vi "ObjectRegistration.vi"(6 "Min Size":i32=40, 7 "Threshold":i32=30, 8 "error in (no error)":errorcluster, 10 "Roy":T1, 11 "Rob":T1) -> (0 "error out":errorcluster, 1 "Alignment quality":dbl, 2 "y displacement":dbl, 3 "x displacement":dbl)   [LabVIEW 2012]
uses:
  <vilib>/vision/Image Controls.llb/IMAQ Image.ctl
panel:
  out "Roy 2":T1(plugin-control)
  out "Roy":T1(plugin-control)
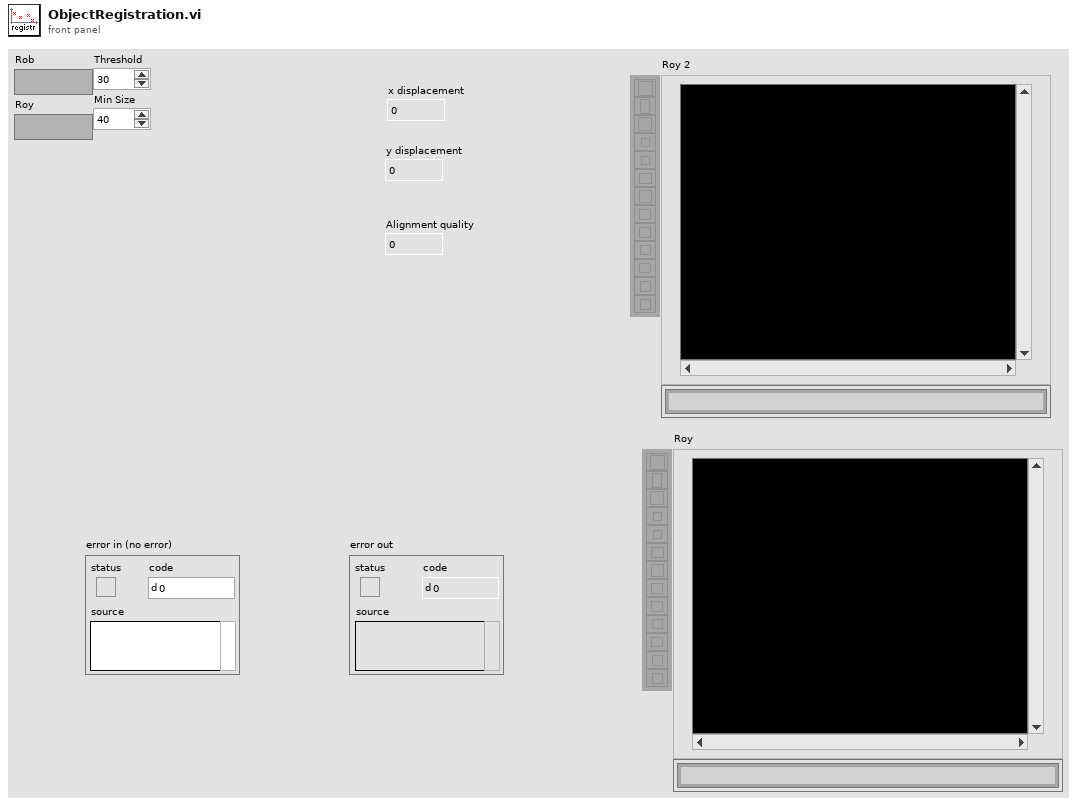
[diagram p1: front panel]
types:
  T1 = typedef "IMAQ Image.ctl" = refnum<image>
  T2 = cluster{"Objects":u16, "Threshold":i32, "Reject Border":bool, "Fill Holes":bool, "Min Object Size":bool, "Min Size":i32, "Max Object Size":bool, "Max Size":i32, "Show Search Area":bool, "Show Center":bool, "Show Bounding Box":bool}
  T3 = cluster{"Object Center":cluster{"X":sgl, "Y":sgl}, "Bounding Box":cluster{"X Left":i32, "Y Top":i32, "X Right":i32, "Y Bottom":i32}, "Area":sgl, "Orientation":sgl, "Aspect Ratio":sgl, "Nb Holes":i32}[]
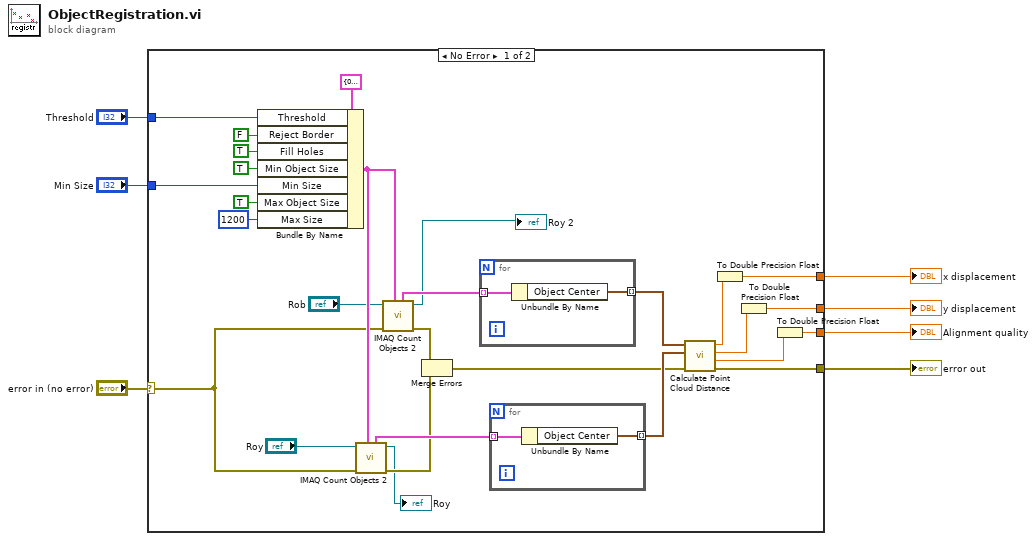
[diagram p0: block diagram]
diagram:
  n1 = case shown="No Error" "error in (no error)" {
    selector: "error in (no error)" -> [w21 w40]
    tunnel: [w20 w40] -> w6
    tunnel: [w16 _] -> w5
    tunnel: [w15 _] -> w4
    tunnel: [w14 _] -> w3
    tunnel: "Threshold" -> [w11 _]
    tunnel: "Min Size" -> [w10 _]
    frame No Error {
      n2 = Bundle By Name(cluster=T2 {"Objects"=0, "Threshold"=128, "Reject Border"=FALSE, "Fill Holes"=FALSE, "Min Object Size"=FALSE, "Min Size"=3, "Max Object Size"=FALSE, "Max Size"=100, "Show Search Area"=FALSE, "Show Center"=TRUE, "Show Bounding Box"=TRUE} ("Settings"), "Threshold"=w11, "Reject Border"=FALSE, "Fill Holes"=TRUE, "Min Object Size"=TRUE, "Min Size"=w10, "Max Object Size"=TRUE, "Max Size"=1200) -> (w31:T2)
      n3 = call "IMAQ Count Objects 2"("Settings"=w31, "error in (no error)"=w21, "Image"="Roy") -> ("error out"=w24:errorcluster, "Image Out"=→"Roy":T1, "Objects"=w29:T3)  [unwired: 4 in, 2 out]
      n4 = call "IMAQ Count Objects 2"("Settings"=w31, "error in (no error)"=w21, "Image"="Rob") -> ("error out"=w23:errorcluster, "Image Out"=→"Roy 2":T1, "Objects"=w30:T3)  [unwired: 4 in, 2 out]
      n5 = Merge Errors(w23, w24) -> (w22:errorcluster)
      n6 = for {
        tunnel: w30 -> [w39] mode=indexing
        tunnel: [w38] -> w28 mode=indexing
        n7 = Unbundle By Name(w39) -> ("Object Center"=w38:cluster{"X":sgl, "Y":sgl})
      }
      n8 = for {
        tunnel: w29 -> [w37] mode=indexing
        tunnel: [w36] -> w27 mode=indexing
        n9 = Unbundle By Name(w37) -> ("Object Center"=w36:cluster{"X":sgl, "Y":sgl})
      }
      n10 = call "Calculate Point Cloud Distance.vi"("error in (no error)"=w22, "Moving point cloud"=w27, "Fixed point cloud"=w28) -> ("error out"=w20:errorcluster, "Alignment quality"=w19:sgl, "y displacement"=w18:sgl, "x displacement"=w17:sgl)  [unwired: 5 in]
      n11 = To Double Precision Float(number=w17) -> (double precision float=w14:dbl)
      n12 = To Double Precision Float(number=w18) -> (double precision float=w15:dbl)
      n13 = To Double Precision Float(number=w19) -> (double precision float=w16:dbl)
    }
    frame Error {
    }
  }
  "x displacement" <- w3
  "y displacement" <- w4
  "Alignment quality" <- w5
  "error out" <- w6
